vi "Pre-Build Action.vi"(6 "Top Level/Always Included VIs":path[](array[path]), 7 "Main Destination Path":path, 9 "Target Name":string, 10 "Build Specification Name":string, 11 "Project Path":path) -> (0 "error out":errorcluster)   [LabVIEW 2020, in "Build Support.lvlib"]
uses:
  <vilib>/Utility/miscctls.llb/LVReplaceWithSaveOptionEnum.ctl
  Build Support.lvlib
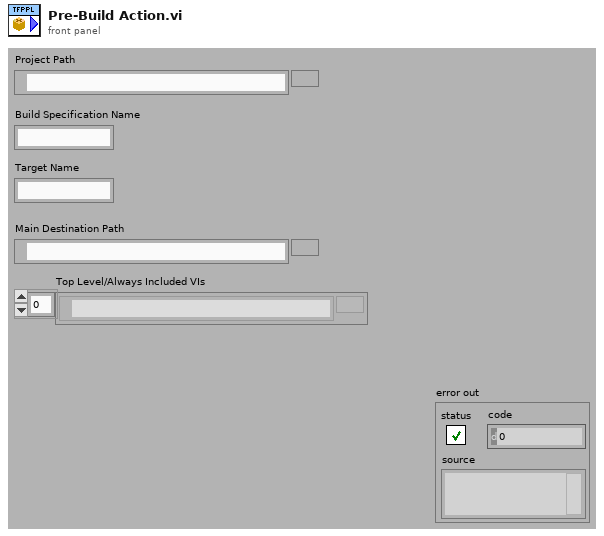
[diagram p1: front panel]
types:
  T1 = typedef "LVReplaceWithSaveOptionEnum.ctl" = enum16{"Save All Without Prompts", "Save All With Prompts", "Do Not Save (Retain In Memory)"}
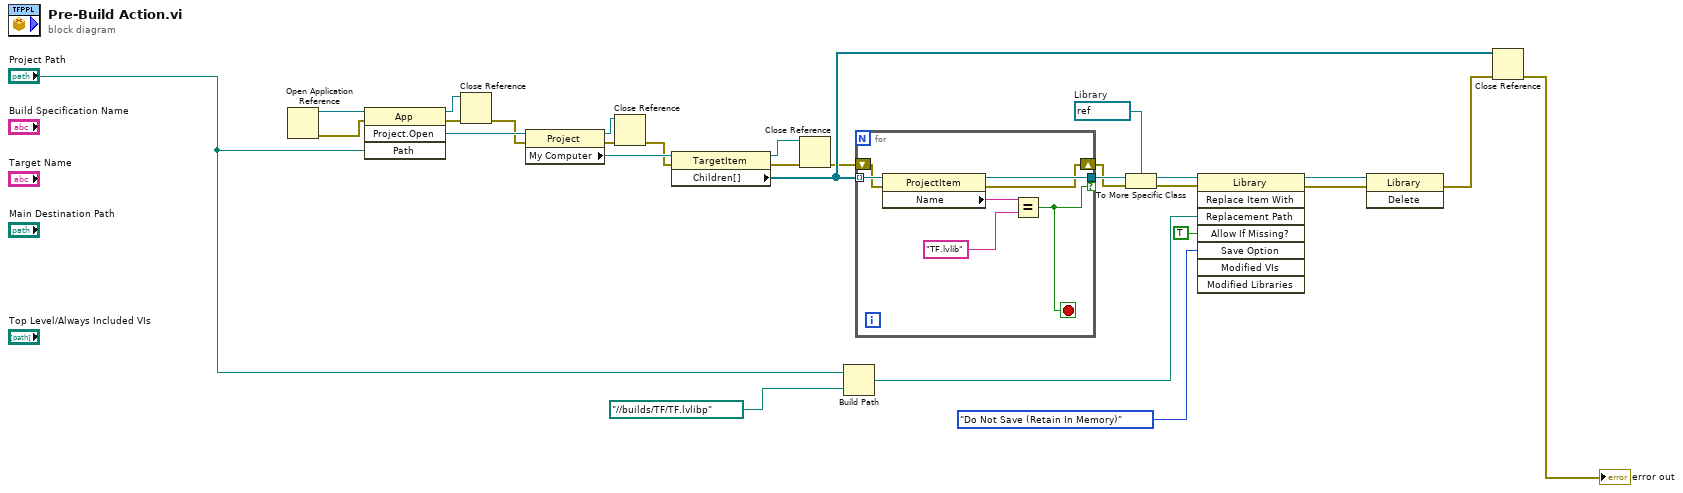
[diagram p0: block diagram]
diagram:
  w23 = refnum<vi> refnum  # Library
  n1 = Open Application Reference() -> (0:w27:errorcluster, 3:w28:refnum<vi>)  [unwired: 4 in]
  n2 = invoke class="App" method="Project.Open"(reference=w28, error in=w27, "Path"="Project Path") -> (reference out=w10:refnum<vi>, error out=w17:errorcluster, "Project:Open"=w26:refnum<vi>)  [unwired: 1 in, 1 out]
  n3 = Close Reference(reference=w10, error in (no error)=w17) -> (error out=w11:errorcluster)
  n4 = property class="Project"(reference=w26, error in=w11) -> (reference out=w8:refnum<vi>, error out=w16:errorcluster, "My Computer"=w25:refnum<vi>)
  n5 = Close Reference(reference=w8, error in (no error)=w16) -> (error out=w9:errorcluster)
  n6 = property class="TargetItem"(reference=w25, error in=w9) -> (reference out=w4:refnum<vi>, error out=w13:errorcluster, "Children[]"=w6:refnum<vi>[])
  n7 = Close Reference(reference=w4, error in (no error)=w13) -> (error out=w5:errorcluster)
  n8 = Build Path(base path="Project Path", name or relative path=path "../../builds/TF/TF.lvlibp") -> (appended path=w19:path)
  n9 = for {
    tunnel: w6 -> [w35] mode=indexing
    tunnel: [w32] -> w24 if=w31
    shift-right: [w29] -> w15
    shift-left: w5 -> [w30]
    stop <- w31 stop-if-true
    n10 = property class="ProjectItem"(reference=w35, error in=w30) -> (reference out=w32:refnum<vi>, error out=w29:errorcluster, "Name"=w34:string)
    n11 = Equal?(x=w34, y="TF.lvlib") -> (x = y?=w31:bool)
  }
  n12 = To More Specific Class(target class=w23, reference=w24, error in=w15) -> (specific class reference=w22:refnum<vi>, error out=w14:errorcluster)
  n13 = invoke class="Library" method="Replace Item With"(reference=w22, error in=w14, "Replacement Path"=w19, "Allow If Missing?"=TRUE, "Save Option"=LVReplaceWithSaveOptionEnum."Do Not Save (Retain In Memory)") -> (reference out=w3:refnum<vi>, error out=w2:errorcluster)  [unwired: 3 in, 6 out]
  n14 = invoke class="Library" method="Delete"(reference=w3, error in=w2) -> (error out=w1:errorcluster)  [unwired: 1 in, 2 out]
  n15 = Close Reference(reference=w6, error in (no error)=w1) -> (error out=→"error out":errorcluster)
